vi "Set RTB Selection Font Size.vi"(8 "Error In":errorcluster, 9 "Font Size (Points)":dbl, 11 ".NET RTB Refnum in":refnum<k24>) -> (0 "Error Out":errorcluster, 3 ".NET RTB Refnum out":refnum<k24>)   [LabVIEW 2021, in "Rich Text Box.lvlib"]
uses:
  Rich Text Box.lvlib
  System.Windows.Forms
  System.Drawing
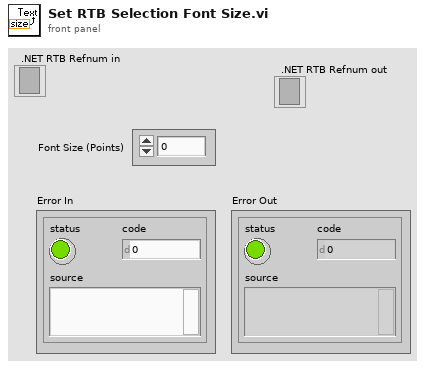
[diagram p1: front panel]
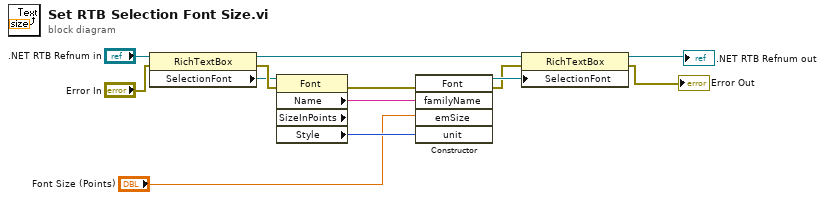
[diagram p0: block diagram]
diagram:
  n1 = property class="RichTextBox"(reference=".NET RTB Refnum in", error in="Error In") -> (reference out=w11:refnum<k24>, error out=w13:errorcluster, "SelectionFont"=w12:refnum<k24>)
  n2 = property class="Font" props=["Name", "SizeInPoints", "Style"](reference=w12, error in=w13) -> (error out=w7:errorcluster, "Name"=w6:string, "Style"=w2:i32)  [unwired: 2 out]
  n3 = constructor class="Font"(error in=w7, "familyName"=w6, "emSize"="Font Size (Points)", "unit"=w2) -> (reference out=w9:refnum<k24>, error out=w8:errorcluster)  [unwired: 2 in, 4 out]
  n4 = property class="RichTextBox"(reference=w11, error in=w8, "SelectionFont"=w9) -> (reference out=→".NET RTB Refnum out":refnum<k24>, error out=→"Error Out":errorcluster)
